vi "Actividad 2 - Lectura.vi"() -> ()   [LabVIEW 2020]
uses:
  <vilib>/httpClient/LabVIEWHTTPClient.lvlib
panel:
  out "Error en Luces":errorcluster
  out "Lateral":bool
  out "Frontal":bool
  out "Temperatura":dbl
  out "body GET":string
  out "headers GET":string
  out "Humedad":dbl
  out "Fecha":string
  in  "stop":bool
  out "Error en Instrumentacion":errorcluster
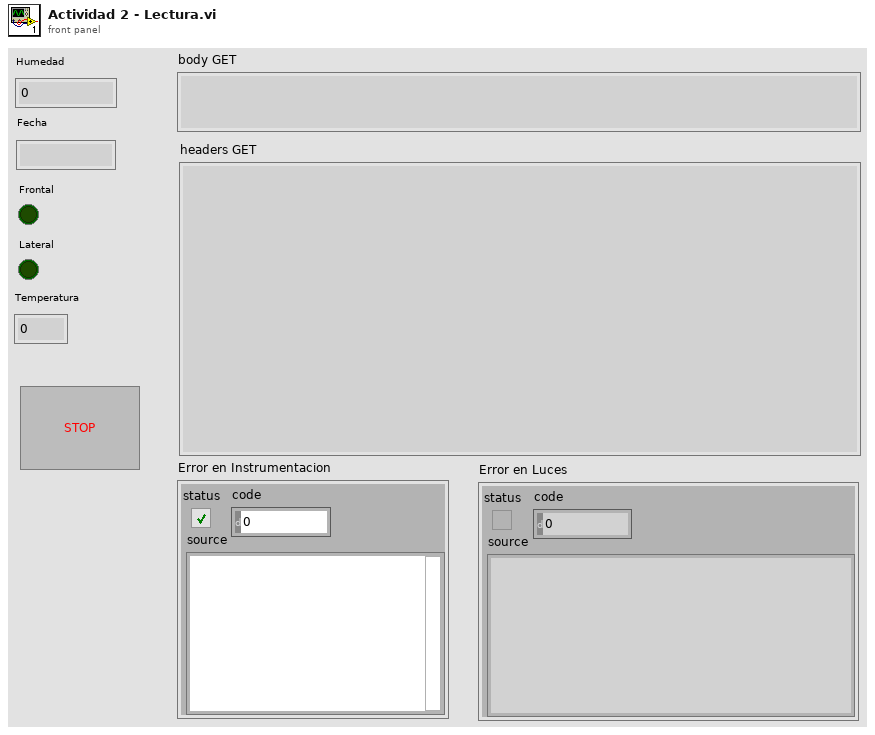
[diagram p1: front panel]
types:
  T1 = cluster{"Humedad":dbl, "Fecha":string, "Temperatura":dbl}
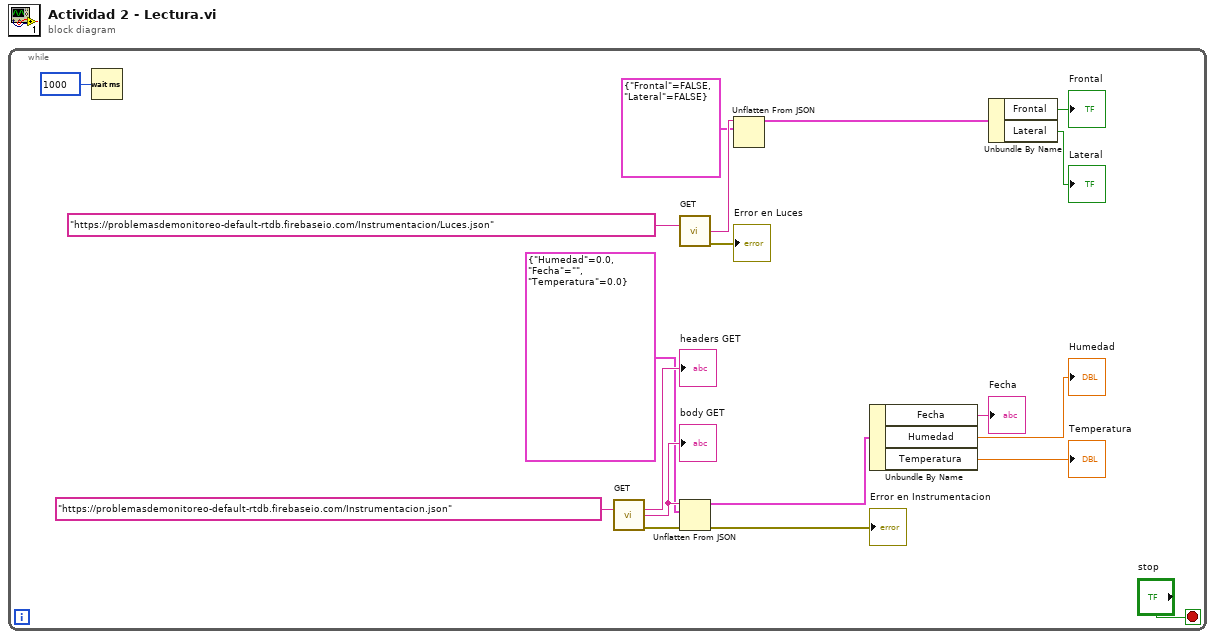
[diagram p0: block diagram]
diagram:
  n1 = while {
    stop <- "stop" stop-if-true
    n2 = Wait (ms)(milliseconds to wait=u32 1000) -> ()  [unwired: 1 out]
    n3 = call <vilib>:"GET.vi"("url"="https://problemasdemonitoreo-default-rtdb.firebaseio.com/Instrumentacion.json") -> ("headers"=→"headers GET":string, "body"=w12:string, "error out"=w17:errorcluster)  [unwired: 11 in, 1 out]
    "body GET" <- w12
    n4 = call <vilib>:"GET.vi"("url"="https://problemasdemonitoreo-default-rtdb.firebaseio.com/Instrumentacion/Luces.json") -> ("body"=w10:string, "error out"=→"Error en Luces":errorcluster)  [unwired: 11 in, 2 out]
    n5 = Unflatten From JSON(JSON string=w12, type and defaults=T1 {"Humedad"=0.0, "Fecha"="", "Temperatura"=0.0}, error in (no error)=w17) -> (value=w16:T1, error out=→"Error en Instrumentacion":errorcluster)  [unwired: 4 in]
    n6 = Unflatten From JSON(JSON string=w10, type and defaults=cluster{"Frontal":bool, "Lateral":bool} {"Frontal"=FALSE, "Lateral"=FALSE}) -> (value=w8:cluster{"Frontal":bool, "Lateral":bool})  [unwired: 5 in, 1 out]
    n7 = Unbundle By Name(w16) -> ("Fecha"=→"Fecha":string, "Humedad"=→"Humedad":dbl, "Temperatura"=→"Temperatura":dbl)
    n8 = Unbundle By Name(w8) -> ("Frontal"=→"Frontal":bool, "Lateral"=→"Lateral":bool)
  }
